vi "Get Parent.vi"(8 "error in (no error)":errorcluster, 11 "Tag_LVOOP in":refnum<class "Tree Tag Class.lvclass">) -> (0 "error out":errorcluster, 1 "Topmost?":bool, 2 "Parent Tag string":string, 3 "Tag_LVOOP out":refnum<class "Tree Tag Class.lvclass">)   [LabVIEW 2012, in "Tree Tools.lvlib" / "Tree Tag Class.lvclass"]
uses:
  Tree Tag Class.lvclass
  Tree Tag Class.lvclass/Tree Tag Class.ctl
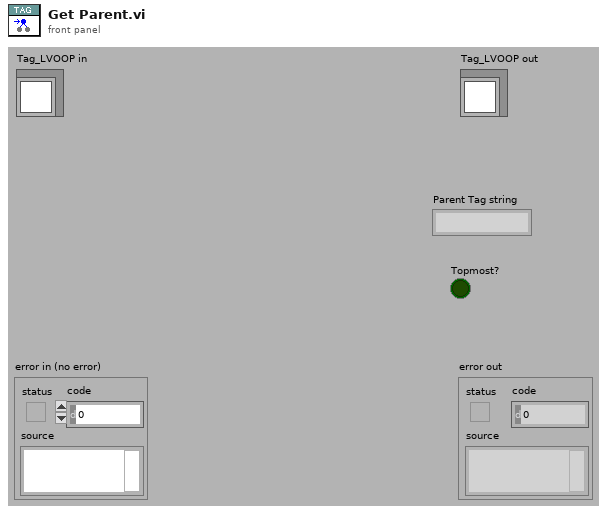
[diagram p1: front panel]
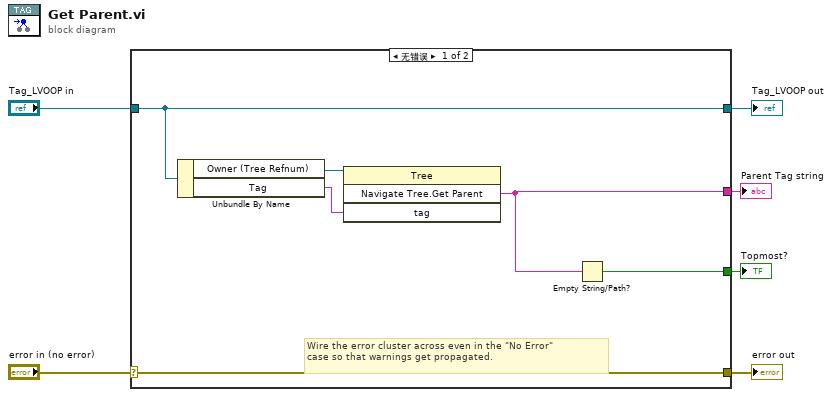
[diagram p0: block diagram]
diagram:
  n1 = case shown="无错误" "error in (no error)" {
    selector: "error in (no error)" -> [w12 w14]
    tunnel: [w12 w14] -> w5
    tunnel: [w11 w13] -> w3
    tunnel: "Tag_LVOOP in" -> [w11 w13]
    tunnel: [w8 _] -> w2
    tunnel: [w7 _] -> w1
    frame No Error {
      # "Wire the error cluster across even in the \"No Error\"\ncase so that warnings get propagated."
      n2 = Unbundle By Name(w11) -> ("Owner (Tree Refnum)"=w10:refnum<vi>, "Tag"=w9:string)
      n3 = invoke class="Tree" method="Navigate Tree.Get Parent"(reference=w10, "tag"=w9) -> ("Navigate Tree:Get Parent"=w8:string)  [unwired: 2 in, 3 out]
      n4 = Empty String/Path?(string/path=w8) -> (empty?=w7:bool)
    }
    frame Error {
    }
  }
  "error out" <- w5
  "Tag_LVOOP out" <- w3
  "Parent Tag string" <- w2
  "Topmost?" <- w1
